vi "GetRefByLabel.vi"(5 "refVI":refnum<vi>, 7 "InsideTab":bool, 8 "error in":errorcluster, 11 "Label":string) -> (0 "error out":errorcluster, 1 "Encontrado?":bool, 3 "Ctl Refnum":refnum<vi>)   [LabVIEW 2018]
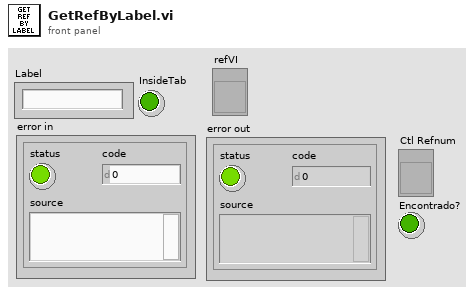
[diagram p1: front panel]
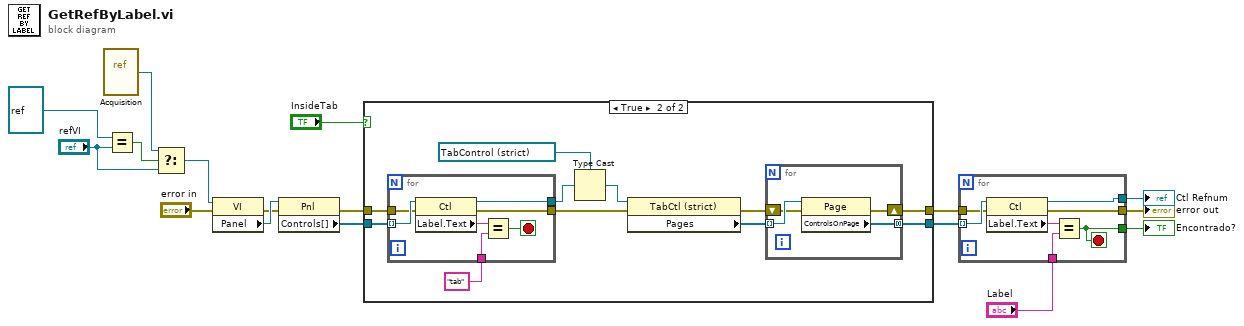
[diagram p0: block diagram]
diagram:
  n1 = vi-ref "Acquisition.vi"() -> (w2:refnum<vi>)
  n2 = Equal?(x=refnum<vi> refnum ("refVI 2"), y="refVI") -> (x = y?=w4:bool)
  n3 = Select(t=w2, s=w4, f="refVI") -> (s? t:f=w1:refnum<vi>)
  n4 = property class="VI"(reference=w1, error in="error in") -> (error out=w13:errorcluster, "Panel"=w17:refnum<vi>)  [unwired: 1 out]
  n5 = property class="Pnl"(reference=w17, error in=w13) -> (error out=w9:errorcluster, "Controls[]"=w7:refnum<vi>[])  [unwired: 1 out]
  n6 = case shown="True" "InsideTab" {
    tunnel: w9 -> [w19 w30]
    tunnel: [w19 w20] -> w8
    tunnel: w7 -> [w18 w29]
    tunnel: [w18 w21] -> w6
    frame False {
    }
    frame True {
      n7 = for {
        tunnel: w29 -> [w41] mode=indexing
        tunnel: "tab" ("Label") -> [w39]
        tunnel: [w38] -> w27
        tunnel: w30 -> [w37]
        tunnel: [w36] -> w24
        stop <- w35 stop-if-true
        n8 = property class="Ctl"(reference=w41, error in=w37) -> (reference out=w38:refnum<vi>, error out=w36:errorcluster, "Label.Text"=w40:string)
        n9 = Equal?(x=w40, y=w39) -> (x = y?=w35:bool)
      }
      n10 = Type Cast(type=refnum<vi> refnum ("tab"), x=w27) -> (*(type *) &x=w25:refnum<vi>)
      n11 = property class="TabCtl (strict)"(reference=w25, error in=w24) -> (error out=w22:errorcluster, "Pages"=w23:refnum<vi>[])  [unwired: 1 out]
      n12 = for {
        tunnel: w23 -> [w34] mode=indexing
        shift-right: [w31] -> w20
        shift-left: w22 -> [w33]
        tunnel: [w32] -> w21 mode=concatenating
        n13 = property class="Page"(reference=w34, error in=w33) -> (error out=w31:errorcluster, "ControlsOnPage"=w32:refnum<vi>[])  [unwired: 1 out]
      }
    }
  }
  n14 = for {
    tunnel: w6 -> [w48] mode=indexing
    tunnel: "Label" -> [w46]
    tunnel: [w45] -> w15
    tunnel: w8 -> [w44]
    tunnel: [w43] -> w12
    tunnel: [w42] -> w11
    stop <- w42 stop-if-true
    n15 = property class="Ctl"(reference=w48, error in=w44) -> (reference out=w45:refnum<vi>, error out=w43:errorcluster, "Label.Text"=w47:string)
    n16 = Equal?(x=w47, y=w46) -> (x = y?=w42:bool)
  }
  "Ctl Refnum" <- w15
  "error out" <- w12
  "Encontrado?" <- w11
